vi "Configure DC Voltage.vi"(0 "VISA resource name":refnum<visa-resource-name>, 1 "Scan List (Empty)":string, 7 "Enable 10M Ohms Input Divider (False)":bool, 11 "error in (no error)":errorcluster) -> (4 "VISA resource name out":refnum<visa-resource-name>, 15 "error out":errorcluster)   [LabVIEW 2020, in "Keithley 27XX.lvlib"]
doc: "This VI configures the Voltage Input Divider for DC Voltage.\nNormally, the input resistance for the 100mVDC, 1VDC, and 10VDC range is >10 GOhms, while the input resistance of the 100VDC and 1000VDC ranges is 10MOhms. However, the input resistance for the three lower DCV ranges can also be set to 10MOhms by enabling the input divider.\n\nWith the input resistance lowered, a more stable 0V reading is achieved with an open input. Also, external devices (such as a high voltage probe) must be terminated by a 10MOhm load.\n\nNote: \n(1) Configure Measurement.vi must be called <B>before</B> configuring the Voltage Input Divider.\n\n(2) This VI will only work when in DC Voltage Measurement mode."
uses:
  <instrlib>/Keithley 27XX/Keithley 27XX.lvlib
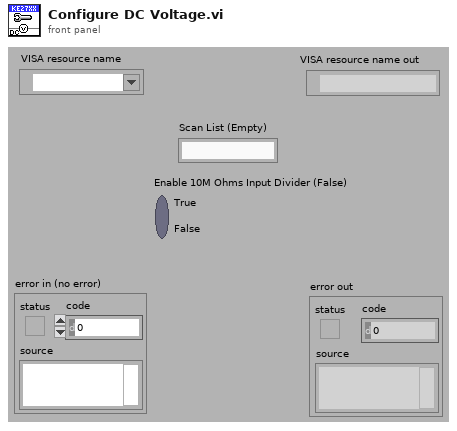
[diagram p1: front panel]
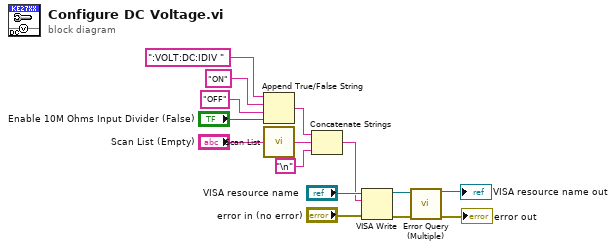
[diagram p0: block diagram]
diagram:
  n1 = Append True/False String(1:"Enable 10M Ohms Input Divider (False)", 2:"OFF" ("false string"), 3:"ON" ("true string"), 4:":VOLT:DC:IDIV " ("string (\"\")")) -> (0:w6:string)
  n2 = call <instrlib>:"Scan List.vi"("Scan List (Empty)"="Scan List (Empty)") -> ("Scan List Out"=w7:string)  [unwired: 14 in]
  n3 = Concatenate Strings(w6, w7, "\n") -> (w8:string)
  n4 = VISA Write(VISA resource name="VISA resource name", write buffer=w8, error in (no error)="error in (no error)") -> (VISA resource name out=w5:refnum<visa-resource-name>, error out=w4:errorcluster)  [unwired: 1 out]
  n5 = call <instrlib>:"Error Query (Multiple).vi"("VISA resource name"=w5, "error in (no error)"=w4) -> ("VISA resource name out"=→"VISA resource name out":refnum<visa-resource-name>, "error out"=→"error out":errorcluster)  [unwired: 10 in, 2 out]
